vi "EstimateStates.vi"(8 "error in (no error)":errorcluster, 10 "Vessel in":refnum<class "Vessel.lvclass">, 11 "Kalman Filter Altitude in":refnum<class "Kalman Filter Altitude.lvclass">) -> (0 "error out":errorcluster, 2 "Vessel out":refnum<class "Vessel.lvclass">, 3 "Kalman Filter Altitude out":refnum<class "Kalman Filter Altitude.lvclass">)   [LabVIEW 2014, in "Observer Library.lvlib" / "Kalman Filter Altitude.lvclass"]
uses:
  Kalman Filter Altitude.lvclass
  ROV/Vessel.lvclass
  Kalman Filter Altitude.lvclass/Kalman Filter Altitude.ctl
  <vilib>/Analysis/Matrix/Numeric/Conversions/Matrix To Array - RM.vi
  <vilib>/imath/engines/lvmath2/RunTimeEngine/IndexRead/NIMS V(S).vi
  <instcachedir>/0/NIMS V(S)_0488751826AF41519A22953C041130DC.lvgen/NIMS V(S)_0488751826AF41519A22953C041130DC_000.vi
  <vilib>/imathl/engines/lvmath/Functions/Error Handling/Create Error.vi
  <vilib>/imath/engines/lvmath2/RunTimeEngine/IndexRead/NIMS V(R2).vi
  <instcachedir>/0/NIMS V(R2)_C76619605A0E4E9F8B2FA9389712AC47.lvgen/NIMS V(R2)_C76619605A0E4E9F8B2FA9389712AC47_000.vi
  <vilib>/imath/engines/lvmath2/RunTimeEngine/ArithmeticOperatorToken/NIMS_ArithmeticOperator_multmx-internal.vi
  <instcachedir>/0/NIMS_ArithmeticOperator_multmx-internal_D7C5C88E94B94895A818D3A8E50A4506.lvgen/NIMS_ArithmeticOperator_multmx-internal_D7C5C88E94B94895A818D3A8E50A4506_004.vi
  <vilib>/imath/engines/lvmath2/RunTimeEngine/ErrorHandling/NIMS_Create Error From Enums.vi
  <vilib>/imath/engines/lvmath2/RunTimeEngine/RangeToken/NIMS_Range_R2 - Integer.vi
  <instcachedir>/0/NIMS_Range_R2 - Integer_2D1304BAF97744E0A293025746CBADFC.lvgen/NIMS_Range_R2 - Integer_2D1304BAF97744E0A293025746CBADFC_000.vi
  <vilib>/imath/engines/lvmath2/RunTimeEngine/CommandStatement/MC_CommandStatement_break.vi
  <vilib>/imath/engines/lvmath2/RunTimeEngine/IndexRead/NIMS M($,S).vi
  <instcachedir>/0/NIMS M($,S)_3E5749BBB62E49528D4765A77F1F6D98.lvgen/NIMS M($,S)_3E5749BBB62E49528D4765A77F1F6D98_001.vi
  <vilib>/imath/engines/lvmath2/RunTimeEngine/IndexReplace/NIMS M($,S)=V.vi
  <instcachedir>/0/NIMS M($,S)=V_9A2C45A15D35467AAEE2181FC06185DD.lvgen/NIMS M($,S)=V_9A2C45A15D35467AAEE2181FC06185DD_000.vi
  <vilib>/imath/engines/lvmath2/RunTimeEngine/ArithmeticOperatorToken/NIMS_ArithmeticOperator_multmx(M,CV)-internal.vi
  <instcachedir>/0/NIMS_ArithmeticOperator_multmx(M,CV)-internal_25C7CE5937BA4322B5BE2717374345EA.lvgen/NIMS_ArithmeticOperator_multmx(M,CV)-internal_25C7CE5937BA4322B5BE2717374345EA_005.vi
  <vilib>/imath/engines/lvmath2/RunTimeEngine/ArithmeticOperatorToken/NIMS_ArithmeticOperator_plus.vi
  <instcachedir>/0/NIMS_ArithmeticOperator_plus_48D6EAACA5D645B09F7EC9C016C2DEA8.lvgen/NIMS_ArithmeticOperator_plus_48D6EAACA5D645B09F7EC9C016C2DEA8_000.vi
  <instcachedir>/0/NIMS V(S)_0488751826AF41519A22953C041130DC.lvgen/NIMS V(S)_0488751826AF41519A22953C041130DC_002.vi
  <vilib>/imath/engines/lvmath2/RunTimeEngine/IndexReplace/NIMS V(S)=S.vi
  <instcachedir>/0/NIMS V(S)=S_2D52C4EC15D8415E870AEE69FB516CCA.lvgen/NIMS V(S)=S_2D52C4EC15D8415E870AEE69FB516CCA_004.vi
  <vilib>/imath/engines/lvmath2/RunTimeEngine/IndexRead/NIMS M(S,S).vi
  <instcachedir>/0/NIMS M(S,S)_AC51E74150A542F7991B9634C66F3096.lvgen/NIMS M(S,S)_AC51E74150A542F7991B9634C66F3096_001.vi
  <instcachedir>/0/NIMS V(S)=S_2D52C4EC15D8415E870AEE69FB516CCA.lvgen/NIMS V(S)=S_2D52C4EC15D8415E870AEE69FB516CCA_001.vi
  <vilib>/imath/engines/lvmath2/RunTimeEngine/BuiltInFunctions/zeros/NIMS_M=zeros(I32,I32).vi
  <vilib>/imath/engines/lvmath2/RunTimeEngine/BuiltInFunctions/zeros/NIMS_V=zeros(I32,I32).vi
  <vilib>/imath/engines/lvmath2/RunTimeEngine/IndexReplace/NIMS M(S,S)=S.vi
  <instcachedir>/0/NIMS M(S,S)=S_43446D47E75543269C90719353EB0EB0.lvgen/NIMS M(S,S)=S_43446D47E75543269C90719353EB0EB0_001.vi
  <vilib>/imath/engines/lvmath2/RunTimeEngine/ArithmeticOperatorToken/NIMS_ArithmeticOperator_multmx.vi
  <instcachedir>/0/NIMS_ArithmeticOperator_multmx_CE3986B82B8C4E94A31593A7EF82383B.lvgen/NIMS_ArithmeticOperator_multmx_CE3986B82B8C4E94A31593A7EF82383B_003.vi
  <vilib>/imath/engines/lvmath2/RunTimeEngine/ArithmeticOperatorToken/NIMS_ArithmeticOperator_multmx(M,CV).vi
  <instcachedir>/0/NIMS_ArithmeticOperator_multmx(M,CV)_787B4652E60B4C52835A7FB23671E425.lvgen/NIMS_ArithmeticOperator_multmx(M,CV)_787B4652E60B4C52835A7FB23671E425_004.vi
  <vilib>/imath/engines/lvmath2/RunTimeEngine/ArithmeticOperatorToken/NIMS_ArithmeticOperator_leftdivmx(C,C).vi
  <instcachedir>/0/NIMS_ArithmeticOperator_leftdivmx(C,C)_9E5ADFA18E304AC7A172DF8AEF23BCA4.lvgen/NIMS_ArithmeticOperator_leftdivmx(C,C)_9E5ADFA18E304AC7A172DF8AEF23BCA4_000.vi
  <vilib>/imath/engines/lvmath2/RunTimeEngine/IndexRead/NIMS M(S).vi
  <instcachedir>/0/NIMS M(S)_B826C018497E4940AE96BD27B540B6FB.lvgen/NIMS M(S)_B826C018497E4940AE96BD27B540B6FB_004.vi
  <vilib>/imath/engines/lvmath2/RunTimeEngine/ArithmeticOperatorToken/NIMS_ArithmeticOperator_multmx(RV,M)-internal.vi
  <instcachedir>/0/NIMS_ArithmeticOperator_multmx(RV,M)-internal_657F30F93C6F47F18CEE3CA5384C5D36.lvgen/NIMS_ArithmeticOperator_multmx(RV,M)-internal_657F30F93C6F47F18CEE3CA5384C5D36_002.vi
  <vilib>/imath/engines/lvmath2/RunTimeEngine/ArithmeticOperatorToken/NIMS_ArithmeticOperator_multmx(RV,CV)-internal.vi
  <instcachedir>/0/NIMS_ArithmeticOperator_multmx(RV,CV)-internal_E181434B092F4BAFA1B7E5F22D537F51.lvgen/NIMS_ArithmeticOperator_multmx(RV,CV)-internal_E181434B092F4BAFA1B7E5F22D537F51_006.vi
  <vilib>/imath/engines/lvmath2/RunTimeEngine/ArithmeticOperatorToken/NIMS_ArithmeticOperator_powermx(M,M).vi
  <instcachedir>/0/NIMS_ArithmeticOperator_multmx_CE3986B82B8C4E94A31593A7EF82383B.lvgen/NIMS_ArithmeticOperator_multmx_CE3986B82B8C4E94A31593A7EF82383B_008.vi
  <instcachedir>/0/NIMS_ArithmeticOperator_plus_48D6EAACA5D645B09F7EC9C016C2DEA8.lvgen/NIMS_ArithmeticOperator_plus_48D6EAACA5D645B09F7EC9C016C2DEA8_002.vi
  <instcachedir>/0/NIMS_ArithmeticOperator_plus_48D6EAACA5D645B09F7EC9C016C2DEA8.lvgen/NIMS_ArithmeticOperator_plus_48D6EAACA5D645B09F7EC9C016C2DEA8_011.vi
  <vilib>/imath/engines/lvmath2/RunTimeEngine/NodeEndStatement/NIMS_NodeEndStatement_Get Scalar.vi
  <instcachedir>/0/NIMS_NodeEndStatement_Get Scalar_62223508BC7F4CFFA0F66459A43A6646.lvgen/NIMS_NodeEndStatement_Get Scalar_62223508BC7F4CFFA0F66459A43A6646_000.vi
  <vilib>/imath/engines/lvmath/Functions/Error Handling/MergeErrorsWrapper.vi
  <vilib>/imath/engines/lvmath2/RunTimeEngine/NodeEndStatement/NIMS_NodeEndStatement_Output.vi
  <instcachedir>/0/NIMS_NodeEndStatement_Output_53EC0D466D134D7ABD903AC30B43404B.lvgen/NIMS_NodeEndStatement_Output_53EC0D466D134D7ABD903AC30B43404B_010.vi
  <instcachedir>/0/NIMS_NodeEndStatement_Output_53EC0D466D134D7ABD903AC30B43404B.lvgen/NIMS_NodeEndStatement_Output_53EC0D466D134D7ABD903AC30B43404B_005.vi
  <instcachedir>/0/NIMS_NodeEndStatement_Output_53EC0D466D134D7ABD903AC30B43404B.lvgen/NIMS_NodeEndStatement_Output_53EC0D466D134D7ABD903AC30B43404B_001.vi
  <vilib>/imath/engines/lvmath2/RunTimeEngine/ErrorHandling/NIMS_Finalize Error.vi
  Supervisor/Supervisor.lvclass
  Sensor/Sensor.lvclass
  <vilib>/Analysis/Matrix/NI_Matrix.lvlib
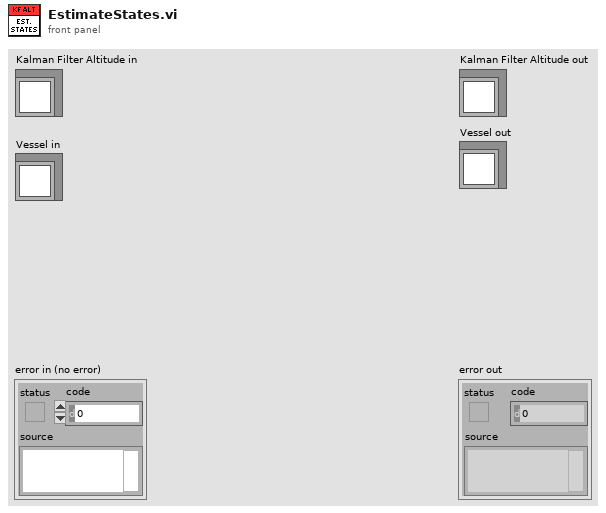
[diagram p1: front panel]
types:
  T1 = cluster{"Altimeter Active":bool, "Beam select":i8, "Value":cluster{"Measured":dbl, "Estimated":dbl, "Desired":dbl, "Previous Desired":dbl, "Approximated":dbl}}
  T2 = cluster{"Measured":cluster{"Eta":dbl[], "Nu":dbl[], "Eta Dot":dbl[], "Nu Dot":dbl[]}, "Estimated":cluster{"Eta":dbl[], "Nu":dbl[], "Eta Dot":dbl[], "Nu Dot":dbl[]}, "Desired":cluster{"Eta":dbl[], "Nu":dbl[], "Eta Dot":dbl[], "Nu Dot":dbl[]}, "Previous Desired":cluster{"Eta":dbl[], "Nu":dbl[], "Eta Dot":dbl[], "Nu Dot":dbl[]}, "tau":dbl[], "Altitude":cluster{"Measured":dbl, "Estimated":dbl, "Desired":dbl, "Previous Desired":dbl, "Approximated":dbl, "grad F":dbl[]}, "rpm":dbl[], "Attitude":cluster{"Theta Measured":dbl[], "Theta Estimated":dbl[], "Omega Measured":dbl[], "Omega Estimated":dbl[], "Gyro Bias":dbl[]}}
  T3 = typedef "NI_Matrix.lvlib/RealMatrix.ctl" = dbl[][]
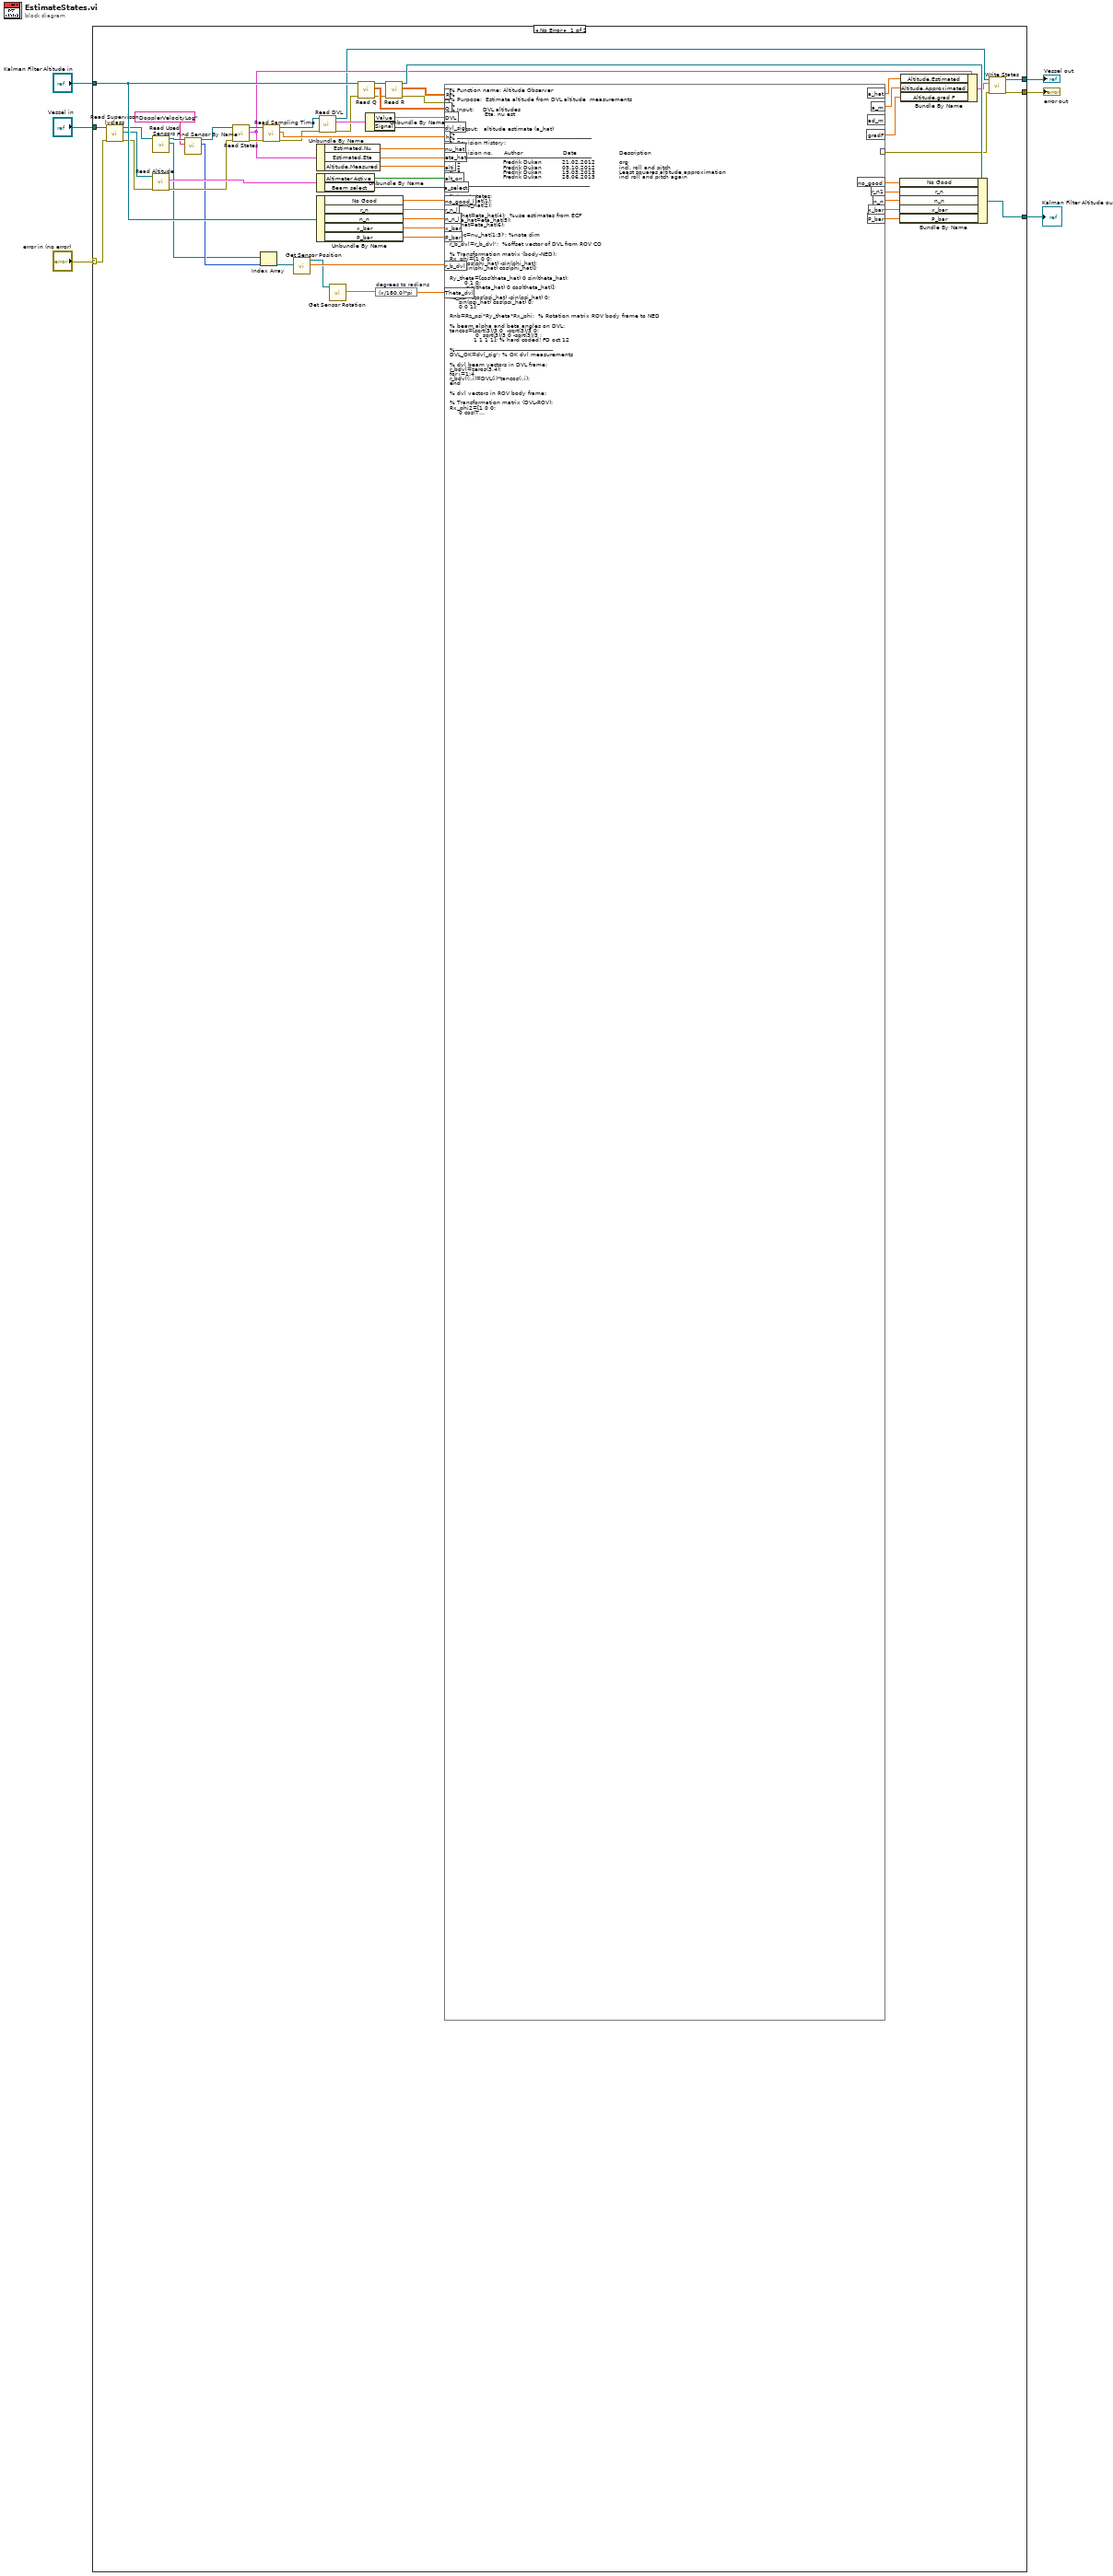
[diagram p0: block diagram]
diagram:
  n1 = case shown="No Error" "error in (no error)" {
    selector: "error in (no error)" -> [w34 w1828]
    tunnel: "Kalman Filter Altitude in" -> [w59 w1830]
    tunnel: "Vessel in" -> [w43 w1829]
    tunnel: [w47 w1830] -> w3
    tunnel: [w22 w1829] -> w2
    tunnel: [w20 w1828] -> w1
    frame No Error {
      n2 = call "Read Supervisor.lvclass.vi"("error in (no error)"=w34, "Vessel in"=w43) -> ("error out"=w33:errorcluster, "Supervisor.lvclass"=w42:refnum<class "Supervisor.lvclass">, "Vessel out"=w17:refnum<class "Vessel.lvclass">)  [unwired: 7 in]
      n3 = call-dynamic "Read Altitude.vi"("error in (no error)"=w33, "Supervisor in"=w42) -> ("error out"=w32:errorcluster, "Altitude"=w41:T1)  [unwired: 7 in, 1 out]
      n4 = call "Read Used Sensors.vi"("Vessel in"=w17) -> ("Used Sensors"=w12:refnum<class "Sensor.lvclass">[], "Vessel out"=w16:refnum<class "Vessel.lvclass">)  [unwired: 8 in, 1 out]
      n5 = call "Find Sensor By Name.vi"("Sensor Name"="DopplerVelocityLog", "Vessel in"=w16) -> ("Sensor Index"=w13:i32, "Vessel out"=w15:refnum<class "Vessel.lvclass">)  [unwired: 7 in, 1 out]
      n6 = call-dynamic "Read States.vi"("error in (no error)"=w32, "Vessel in"=w15) -> ("error out"=w31:errorcluster, "States"=w26:T2, "Vessel out"=w38:refnum<class "Vessel.lvclass">)  [unwired: 7 in]
      n7 = Index Array(array=w12, index=w13) -> (element=w11:refnum<class "Sensor.lvclass">)
      n8 = call-dynamic "Read Sampling Time.vi"("error in (no error)"=w31, "Vessel in"=w38) -> ("error out"=w30:errorcluster, "Sampling Time"=w36:dbl, "Vessel out"=w37:refnum<class "Vessel.lvclass">)  [unwired: 7 in]
      n9 = call-dynamic "Get Sensor Position.vi"("Sensor in"=w11) -> ("Sensor Position"=w10:dbl[], "Sensor out"=w9:refnum<class "Sensor.lvclass">)  [unwired: 8 in, 1 out]
      n10 = Unbundle By Name(w26) -> ("Estimated.Nu"=w60:dbl[], "Estimated.Eta"=w61:dbl[], "Altitude.Measured"=w35:dbl)
      n11 = Unbundle By Name(w41) -> ("Altimeter Active"=w40:bool, "Beam select"=w39:i8)
      n12 = Unbundle By Name(w59) -> ("No Good"=w58:dbl, "r_n"=w57:dbl[], "n_n"=w56:dbl[], "x_bar"=w55:dbl, "P_bar"=w54:dbl)
      n13 = call-dynamic "Read DVL.vi"("error in (no error)"=w30, "Vessel in"=w37) -> ("error out"=w29:errorcluster, "DVL"=w46:cluster{"Value":dbl[], "Signal":i32[]}, "Vessel out"=w23:refnum<class "Vessel.lvclass">)  [unwired: 7 in]
      n14 = call-dynamic "Get Sensor Rotation.vi"("Sensor in"=w9) -> ("Sensor Rotation"=w7:dbl[])  [unwired: 8 in, 2 out]
      n15 = call-dynamic "Read Q.vi"("error in (no error)"=w29, "Kalman Filter in"=w59) -> ("error out"=w28:errorcluster, "Real Matrix"=w63:T3, "Kalman Filter out"=w62:refnum<class "Kalman Filter Altitude.lvclass">)  [unwired: 7 in]
      n16 = Unbundle By Name(w46) -> ("Value"=w44:dbl[], "Signal"=w45:i32[])
      n17 = expression code="(x/180.0)*pi" "degrees to radians"(w7) -> (w8:dbl[])
      n18 = call-dynamic "Read R.vi"("error in (no error)"=w28, "Kalman Filter in"=w62) -> ("error out"=w27:errorcluster, "Real Matrix"=w64:T3, "Kalman Filter out"=w53:refnum<class "Kalman Filter Altitude.lvclass">)  [unwired: 7 in]
      n19 = mathscript code="% Function name: Altitude Observer\n%\n% Purpose:  Estimate altitude from DVL altitude  measurements\n%\n% Input:     DVL altitudes\n%                Eta, nu est\n%                \n%\n% Output:   altitude estimate (a_hat)\n%\n% -------------------------------------------------------------------------\n% Revision History:\n%\n% Revision no.      Author                      Date                       Description\n%--------------------------------------------------------------------------\n% 1                       Fredrik Dukan           21.02.2012             org \n% 2                       Fredrik Dukan           05.10.2012             incl. roll and pitch         \n% 3                       Fredrik Dukan           15.03.2013             Least squares altitude approximation \n% 4                       Fredrik Dukan           28.06.2013             incl roll and pitch again\n\n%-------------------------------------------------------------------------\n\n% Input states:\n%u=nu_hat(1);\n%v=nu_hat(2);\n\nphi_hat=eta_hat(4);  %use estimates from ECF\ntheta_hat=eta_hat(5);\npsi_hat=eta_hat(6);\n\nv_vec=nu_hat(1:3)'; %note dim\n\nr_b_dvl=r_b_dvl';  %offset vector of DVL from ROV CO\n\n% Transformation matrix (body-NED):\nRx_phi=[1 0 0;\n     0 cos(phi_hat) -sin(phi_hat);\n     0 sin(phi_hat) cos(phi_hat)];\n\nRy_theta=[cos(theta_hat) 0 sin(theta_hat);\n        0 1 0;\n        -sin(theta_hat) 0 cos(theta_hat)];\n \nRz_psi=[cos(psi_hat) -sin(psi_hat) 0;\n     sin(psi_hat) cos(psi_hat) 0;\n     0 0 1]; \n \nRnb=Rz_psi*Ry_theta*Rx_phi;  % Rotation matrix ROV body frame to NED\n\n% beam alpha and beta angles on DVL:\ntancos=[sqrt(3)/3 0  -sqrt(3)/3 0;\n              0  sqrt(3)/3 0 -sqrt(3)/3 ;\n             1 1 1 1]; % hard coded! FD oct 12\n\n%-----------------------------------------------------\nDVL_OK=dvl_sig'; % OK dvl measurements\n\n% dvl beam vectors in DVL frame:\nr_bdvl=zeros(3,4);\nfor i=1:4\nr_bdvl(:,i)=DVL(i)*tancos(:,i);\nend\n\n% dvl vectors in ROV body frame:\n\n% Transformation matrix (DVL-ROV):\nRx_phi2=[1 0 0;\n     0 cos(Theta_dvl(1)) -sin(Theta_dvl(1));\n     0 sin(Theta_dvl(1)) cos(Theta_dvl(1))];\n\nRy_theta2=[cos(Theta_dvl(2)) 0 sin(Theta_dvl(2));\n        0 1 0;\n        -sin(Theta_dvl(2)) 0 cos(Theta_dvl(2))];\n \nRz_psi2=[cos(Theta_dvl(3)) -sin(Theta_dvl(3)) 0;\n     sin(Theta_dvl(3)) cos(Theta_dvl(3)) 0;\n     0 0 1]; \n \nRnb_dvl=Rz_psi2*Ry_theta2*Rx_phi2;  % Rotation matrix ROV body frame to NED (NOTE: need only calc this once)\n \nr_brov=zeros(3,4);\nfor i=1:4\nr_brov(:,i)=Rnb_dvl*r_bdvl(:,i)+r_b_dvl;\nend\n\n% dvl vectors in NED frame: \nr_n=zeros(3,4);\nfor i=1:4\nr_n(:,i)=Rnb*r_brov(:,i);\nend\n\n% find good dvl measurements:\nnok=0;\ngood=zeros(1,4);\nfor i=1:4\n  nok=nok+DVL_OK(i);\n  if DVL_OK(i)==1\n  good(nok)=i;\n  end\nend\n\n%% Calculate approximated sea floor -----------------------------------\nif nok>=3 % at least 3 good DVL measurements..\n\nA=zeros(nok,3); % see eq. (15) in FD alt paper\nb=zeros(nok,1); % ==\n \n% Set up linear system:\nfor i=1:nok\n   A(i,1)=1;\n   A(i,2)=r_n(1,good(i));   %\n   A(i,3)=r_n(2,good(i));   %\n   b(i)=r_n(3,good(i));      %\nend\n\nATA=A'*A;\nATb=A'*b;\n\n%solve system\nabc=ATA\\ATb;\n\nno_good=0;\nelseif nok==2\nabc=zeros(3,1);\nabc(1)=(r_n(3,good(1))+r_n(3,good(2)))/2;\nabc(2)=0;\nabc(3)=0;\nno_good=0;\n\nelseif nok==1 %only 1 dvl beam\nabc(1)=r_n(3,good(1));\nabc(2)=0;\nabc(3)=0;\nno_good=0;\n\nelse % no good dvl measurements\nabc(1)=0;\nabc(2)=0;\nabc(3)=0;\nno_good=no_good_l+1;\nend\n\na_m=abc(1);  % approximated altitude\n\ngradF=zeros(1,3);\ngradF(1)=abc(2);\ngradF(2)=abc(3);\ngradF(3)=-1;  % approximated gradient vector\n\nad_m=gradF*Rnb*v_vec; % approximated altitude rate of change (mean)\n\n%% Kalman Filter for altitude estimation: -----------------------------\n\nPHI=1;\nDELTA=h; %h is time step [s]\nGAMMA=-h;\n\nH=1;  %Note: should be updated for available measurements.\n\n% use approximated altitude or sonar altitude:\nif ~alt_on\ny=a_m;    %scalar KF\nelse\ny=alti;    %scalar KF\nend\n\nu_e=ad_m;\nI=1; %eye(size(DELTA,1));\n\n% Gain:\n    K=P_bar*H'*[H*P_bar*H'+R]^-1;\n% Corrector:\n    P_hat=[I-K*H]*P_bar*[I-K*H]'+K*R*K';\n    x_hat=x_bar+K*[y-H*x_bar];\n%Predictor:\n    x_bar=PHI*x_hat+DELTA*u_e; \n    P_bar=PHI*P_hat*PHI'+GAMMA*Q*GAMMA';\n\n% output of observer:\na_hat=x_hat;\n\n%%------------------------------------------------------------------\nr_n1=r_n(:,1); % bare vas:---\nn_n=gradF';"("??"=w27, "DVL"=w44, "dvl_sig"=w45, "eta_hat"=w61, "nu_hat"=w60, "h"=w36, "x_bar"=w55, "P_bar"=w54, "R"=w64, "Q"=w63, "alti"=w35, "alt_on"=w40, "a_select"=w39, "r_n_l"=w57, "n_n_l"=w56, "no_good_l"=w58, "r_b_dvl"=w10, "Theta_dvl"=w8) -> ("??"=w21:errorcluster, "P_bar"=w48:dbl, "x_bar"=w49:dbl, "a_hat"=w25:dbl, "gradF"=w18:dbl[], "a_m"=w19:cdb, "n_n"=w50:dbl[], "r_n1"=w51:dbl[], "no_good"=w52:dbl)  [unwired: 1 out]
      n20 = Bundle By Name(cluster=w53, "No Good"=w52, "r_n"=w51, "n_n"=w50, "x_bar"=w49, "P_bar"=w48) -> (w47:refnum<class "Kalman Filter Altitude.lvclass">)
      n21 = Bundle By Name(cluster=w26, "Altitude.Estimated"=w25, "Altitude.Approximated"=w19, "Altitude.grad F"=w18) -> (w24:T2)
      n22 = call-dynamic "Write States.vi"("error in (no error)"=w21, "States"=w24, "Vessel in"=w23) -> ("error out"=w20:errorcluster, "Vessel out"=w22:refnum<class "Vessel.lvclass">)  [unwired: 7 in]
    }
    frame Error {
    }
  }
  "error out" <- w1
  "Kalman Filter Altitude out" <- w3
  "Vessel out" <- w2
